vi "Sigma.vi"(6 "Size subgroup":i32=5, 7 "Type sigma (stand dev)":enum16{"stand dev", "R/d2", "tau"}(ring), 8 "Error In":errorcluster, 9 "Low limit":dbl, 10 "High limit":dbl, 11 "Data":dbl[](array[numeric])) -> (0 "Error Out":errorcluster, 2 "Sigma":dbl, 3 "Mean":dbl)   [LabVIEW 2019, in "Tools.lvlib"]
uses:
  Tools.lvlib
  <vilib>/Analysis/NI_AALBase.lvlib
panel:
  in  "d2":dbl[](array[numeric])=[1.128, 1.693, 2.059, 2.326, 2.534, 2.704, 2.847, 2.97, 3.078, 3.173, 3.258, 3.336, 3.407, 3.472, 3.532, 3.588, 3.64, 3.689, 3.735, 3.778, 3.819, 3.858, 3.895, 3.931]
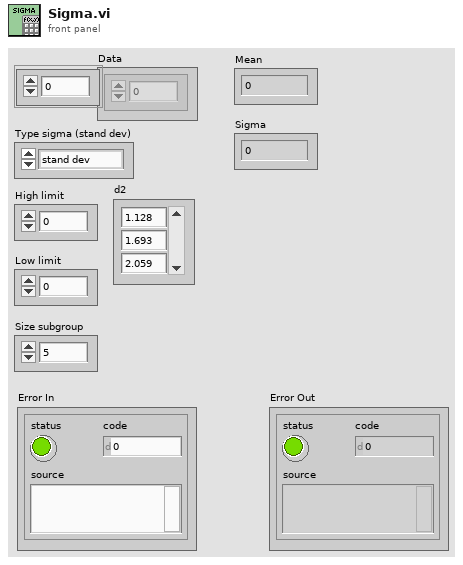
[diagram p1: front panel]
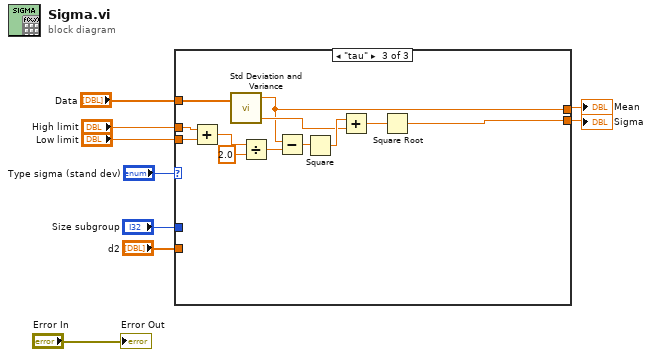
[diagram p0: block diagram]
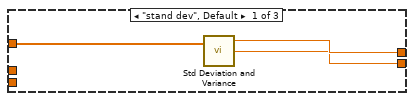
[diagram p2: hidden frame]
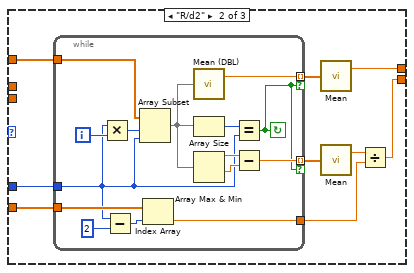
[diagram p3: hidden frame]
diagram:
  n1 = case shown="\"tau\"" "Type sigma (stand dev)" {
    tunnel: "Data" -> [w11 w21 w45]
    tunnel: [w12 w15 w40] -> w7
    tunnel: [w10 w18 w41] -> w8
    tunnel: "Low limit" -> [_ _ w47]
    tunnel: "High limit" -> [_ _ w48]
    tunnel: "Size subgroup" -> [_ w20 _]
    tunnel: "d2" -> [_ w19 _]
    frame "stand dev", Default {
      n2 = call <vilib>:"Std Deviation and Variance.vi"("X"=w11) -> ("mean"=w12:dbl, "standard deviation"=w10:dbl)  [unwired: 1 in, 1 out]
    }
    frame "R/d2" {
      n3 = while {
        tunnel: w21 -> [w32]
        tunnel: [w36] -> w16 mode=indexing if=w27
        tunnel: [w35] -> w14 mode=indexing if=w27
        tunnel: w20 -> [w25]
        tunnel: w19 -> [w26]
        tunnel: [w22] -> w17
        i -> [w31]
        stop <- w27 continue-if-true
        n4 = Multiply(x=w25, y=w31) -> (x*y=w30:i32)
        n5 = Subtract(x=w25, y=2) -> (x-y=w24:i32)
        n6 = Array Subset(array=w32, index=w30, length=w25) -> (w28:dbl[])
        n7 = Index Array(array=w26, index=w24) -> (element=w22:dbl)
        n8 = call <vilib>:"Mean (DBL).vi"("X"=w28) -> ("mean"=w36:dbl)  [unwired: 1 out]
        n9 = Array Size(array=w28) -> (size(s)=w29:i32)
        n10 = Array Max & Min(array=w28) -> (max value=w34:dbl, min value=w33:dbl)  [unwired: 2 out]
        n11 = Equal?(x=w29, y=w25) -> (x = y?=w27:bool)
        n12 = Subtract(x=w34, y=w33) -> (x-y=w35:dbl)
      }
      n13 = call-poly <vilib>:"Mean.vi"("X"=w16) -> ("mean"=w15:dbl)  [unwired: 1 out]
      n14 = call-poly <vilib>:"Mean.vi"("X"=w14) -> ("mean"=w13:dbl)  [unwired: 1 out]
      n15 = Divide(x=w13, y=w17) -> (x/y=w18:dbl)
    }
    frame "tau" {
      n16 = Add(x=w48, y=w47) -> (x+y=w38:dbl)
      n17 = call <vilib>:"Std Deviation and Variance.vi"("X"=w45) -> ("mean"=w40:dbl, "variance"=w43:dbl)  [unwired: 1 in, 1 out]
      n18 = Divide(x=w38, y=2.0) -> (x/y=w39:dbl)
      n19 = Subtract(x=w40, y=w39) -> (x-y=w46:dbl)
      n20 = Square(x=w46) -> (x^2=w44:dbl)
      n21 = Add(x=w44, y=w43) -> (x+y=w42:dbl)
      n22 = Square Root(x=w42) -> (sqrt(x)=w41:dbl)
    }
  }
  "Mean" <- w7
  "Sigma" <- w8
  "Error Out" <- "Error In"
